vi "DecayAnalysis.vi"() -> ()   [LabVIEW 2015]
uses:
  <vilib>/gmath/SpecialFunctions.llb/Factorial.vi
  <vilib>/Utility/file.llb/Read Delimited Spreadsheet (DBL).vi
  <vilib>/imath/engines/lvmath2/RunTimeEngine/Managers/WorkSpace/UID Generator.vi
  <vilib>/imath/engines/lvmath2/RunTimeEngine/BuiltInFunctions/length/NIMS_length(GM).vi
  <instcachedir>/0/NIMS_length(GM)_47CEC356FCE0482D9BA47DC61C99F2C7.lvgen/NIMS_length(GM)_47CEC356FCE0482D9BA47DC61C99F2C7_000.vi
  <vilib>/imath/engines/lvmath2/RunTimeEngine/RangeToken/NIMS_Range.vi
  <instcachedir>/0/NIMS_Range_D919CC09935940E88F755EC1C6F49AC1.lvgen/NIMS_Range_D919CC09935940E88F755EC1C6F49AC1_001.vi
  <vilib>/imath/engines/lvmath2/RunTimeEngine/RunTimeType/NIMS_RunTimeType_From StrictType (excl LVString).vi
  <instcachedir>/0/NIMS_RunTimeType_From StrictType (excl LVString)_EB1C38A9BC5048DA9ABDA8F781E54D21.lvgen/NIMS_RunTimeType_From StrictType (excl LVString)_EB1C38A9BC5048DA9ABDA8F781E54D21_000.vi
  <vilib>/imathl/engines/lvmath/Functions/Error Handling/Create Error.vi
  <vilib>/imath/engines/lvmath2/RunTimeEngine/LocalVariableDefStatement/MC_LocalVariableDefStatement_Display.vi
  <vilib>/imath/engines/lvmath2/RunTimeEngine/Managers/SymbolTable/Clear UID.vi
  <vilib>/imath/engines/lvmath2/RunTimeEngine/NodeEndStatement/NIMS_NodeEndStatement_Output.vi
  <instcachedir>/0/NIMS_NodeEndStatement_Output_53EC0D466D134D7ABD903AC30B43404B.lvgen/NIMS_NodeEndStatement_Output_53EC0D466D134D7ABD903AC30B43404B_004.vi
  <vilib>/imath/engines/lvmath2/RunTimeEngine/ErrorHandling/NIMS_Finalize Error.vi
  <instcachedir>/0/NIMS_NodeEndStatement_Output_53EC0D466D134D7ABD903AC30B43404B.lvgen/NIMS_NodeEndStatement_Output_53EC0D466D134D7ABD903AC30B43404B_005.vi
  <vilib>/imath/engines/lvmath2/RunTimeEngine/Managers/SymbolTable/NIMS_WorkSpace.lvlib
  <vilib>/Analysis/NI_AALBase.lvlib
  <vilib>/gmath/NI_Gmath.lvlib
panel:
  out "XY Graph 2":cluster{"X Values":dbl[], "y":dbl[]}[](graph)=[{"X Values"=[1.8, 5.4, 9.0, 12.6, 16.2, 19.8, 23.4, 27.0, 30.6, 34.2, 37.8, 41.4, 45.0, 48.6, 52.2, 55.8, 59.4, 63.0, 66.6, 70.2], "y"=[1.0, 0.0, 0.0, 0.0, 0.0, 0.0, 0.0, 0.0, 0.0, 3.0, 11.0, 31.0, 36.0, 61.0, 51.0, 51.0, 35.0, 12.0, 6.0, 3.0]}, {"X Values"=[30.0, 31.0, 32.0, 33.0, 34.0, 35.0, 36.0, 37.0, 38.0, 39.0, 40.0, 41.0, 42.0, 43.0, 44.0, 45.0, 46.0, 47.0, 48.0, 49.0, 50.0, 51.0, 52.0, 53.0, 54.0, 55.0, 56.0, 57.0, 58.0, 59.0, 60.0, 61.0, 62.0, 63.0, 64.0, 65.0, 66.0, 67.0, 68.0, 69.0, 70.0, 71.0, 72.0, 73.0, 74.0, 75.0], "y"=[0.2988606313000329, 0.5013146073419906, 0.8146362369307348, 1.2836692218302488, 1.9632588098580277, 2.916841660360498, 4.213215731631831, 5.921276163374466, 8.102798960407162, 10.80373194720955, 14.044851531372414, 17.81298243003331, 22.054168722898382, 26.670157525365486, 31.519277075431937, 36.422275731610235, 41.17300734877679, 45.55311451354027, 49.349207389668635, 52.370587433934055, 54.46541093129141, 55.53336016523831, 55.53336016523831, 54.485560916837585, 52.467577179176935, 49.605709333040004, 46.062444380680006, 42.02187908412913, 37.67478814439164, 33.20489802556551, 28.777578288823435, 24.53170608227572, 20.57497929481189, 16.982522592543145, 13.798299606441311, 11.03863968515305, 8.697110054969068, 6.749995863558084, 5.161761542720885, 3.8900231916157404, 2.889731513771693, 2.1164230805088455, 1.5285277803674993, 1.0888143093028764, 0.7651127578885076, 0.5304781788026988]}]
  in  "file path (dialog if empty) 2":path=path "C:/Users/jamism2/Desktop/PHYS434jampet/week8/constant.txt"
  out "Results":T1={"Array[0]"=67.95538478705842, "Decay Time  (s)"=137.37711750375104, "Array[2]"=-5.05656305145657, "Array[3]"=0.0, "Array[4]"=0.0, "Array[5]"=0.0, "Array[6]"=0.0, "Array[7]"=0.0, "Array[8]"=0.0}
  in  "file path (dialog if empty)":path=path "C:/Users/jamism2/Desktop/PHYS434jampet/week8/decay.txt"
  out "XY Graph":cluster{"Array":dbl[], "all rows":dbl[]}[](graph)=[{"Array"=[0.0, 1.0, 2.0, 3.0, 4.0, 5.0, 6.0, 7.0, 8.0, 9.0, 10.0, 11.0, 12.0, 13.0, 14.0, 15.0, 16.0, 17.0, 18.0, 19.0, 20.0, 21.0, 22.0, 23.0, 24.0, 25.0, 26.0, 27.0, 28.0, 29.0, 30.0, 31.0, 32.0, 33.0, 34.0, 35.0, 36.0, 37.0, 38.0, 39.0, 40.0, 41.0, 42.0, 43.0, 44.0, 45.0, 46.0, 47.0, 48.0, 49.0, 50.0, 51.0, 52.0, 53.0, 54.0, 55.0, 56.0, 57.0, 58.0, 59.0, 60.0, 61.0, 62.0, 63.0, 64.0, 65.0, 66.0, 67.0, 68.0, 69.0, 70.0, 71.0, 72.0, 73.0, 74.0, 75.0, 76.0, 77.0, 78.0, 79.0, 80.0, 81.0, 82.0, 83.0, 84.0, 85.0, 86.0, 87.0, 88.0, 89.0, 90.0, 91.0, 92.0, 93.0, 94.0, 95.0, 96.0, 97.0, 98.0, 99.0, 100.0, 101.0, 102.0, 103.0, 104.0, 105.0, 106.0, 107.0, 108.0, 109.0, 110.0, 111.0, 112.0, 113.0, 114.0, 115.0, 116.0, 117.0, 118.0, 119.0, 120.0, 121.0, 122.0, 123.0, 124.0, 125.0, 126.0, 127.0, 128.0, 129.0, 130.0, 131.0, 132.0, 133.0, 134.0, 135.0, 136.0, 137.0, 138.0, 139.0, 140.0, 141.0, 142.0, 143.0, 144.0, 145.0, 146.0, 147.0, 148.0, 149.0, 150.0, 151.0, 152.0, 153.0, 154.0, 155.0, 156.0, 157.0, 158.0, 159.0, 160.0, 161.0, 162.0, 163.0, 164.0, 165.0, 166.0, 167.0, 168.0, 169.0, 170.0, 171.0, 172.0, 173.0, 174.0, 175.0, 176.0, 177.0, 178.0, 179.0, 180.0, 181.0, 182.0, 183.0, 184.0, 185.0, 186.0, 187.0, 188.0, 189.0, 190.0, 191.0, 192.0, 193.0, 194.0, 195.0, 196.0, 197.0, 198.0, 199.0, 200.0, 201.0, 202.0, 203.0, 204.0, 205.0, 206.0, 207.0, 208.0, 209.0, 210.0, 211.0, 212.0, 213.0, 214.0, 215.0, 216.0, 217.0, 218.0, 219.0, 220.0, 221.0, 222.0, 223.0, 224.0, 225.0, 226.0, 227.0, 228.0, 229.0, 230.0, 231.0, 232.0, 233.0, 234.0, 235.0, 236.0, 237.0, 238.0, 239.0, 240.0, 241.0, 242.0, 243.0, 244.0, 245.0, 246.0, 247.0, 248.0, 249.0, 250.0, 251.0, 252.0, 253.0, 254.0, 255.0, 256.0, 257.0, 258.0, 259.0, 260.0, 261.0, 262.0, 263.0, 264.0, 265.0, 266.0, 267.0, 268.0, 269.0, 270.0, 271.0, 272.0, 273.0, 274.0, 275.0, 276.0, 277.0, 278.0, 279.0, 280.0, 281.0, 282.0, 283.0, 284.0, 285.0, 286.0, 287.0, 288.0, 289.0, 290.0, 291.0, 292.0, 293.0, 294.0, 295.0, 296.0, 297.0, 298.0, 299.0, 300.0, 301.0], "all rows"=[0.0, 47.0, 44.0, 50.0, 68.0, 51.0, 62.0, 72.0, 48.0, 45.0, 45.0, 74.0, 55.0, 72.0, 61.0, 65.0, 59.0, 55.0, 73.0, 56.0, 57.0, 63.0, 54.0, 59.0, 53.0, 55.0, 54.0, 50.0, 53.0, 50.0, 43.0, 50.0, 47.0, 45.0, 43.0, 52.0, 68.0, 50.0, 40.0, 55.0, 62.0, 42.0, 53.0, 55.0, 60.0, 50.0, 51.0, 42.0, 48.0, 35.0, 51.0, 33.0, 35.0, 43.0, 43.0, 54.0, 44.0, 35.0, 31.0, 42.0, 39.0, 46.0, 39.0, 42.0, 41.0, 52.0, 34.0, 42.0, 45.0, 40.0, 50.0, 38.0, 42.0, 30.0, 48.0, 34.0, 27.0, 36.0, 39.0, 32.0, 33.0, 36.0, 26.0, 31.0, 35.0, 25.0, 23.0, 25.0, 38.0, 26.0, 32.0, 34.0, 31.0, 25.0, 36.0, 27.0, 28.0, 26.0, 28.0, 34.0, 30.0, 28.0, 23.0, 30.0, 19.0, 29.0, 17.0, 16.0, 19.0, 24.0, 22.0, 19.0, 27.0, 18.0, 20.0, 23.0, 28.0, 29.0, 28.0, 29.0, 31.0, 21.0, 25.0, 28.0, 26.0, 19.0, 22.0, 27.0, 21.0, 14.0, 9.0, 20.0, 21.0, 15.0, 15.0, 18.0, 15.0, 18.0, 14.0, 14.0, 13.0, 13.0, 12.0, 26.0, 21.0, 26.0, 21.0, 12.0, 7.0, 20.0, 11.0, 18.0, 12.0, 12.0, 16.0, 12.0, 19.0, 13.0, 9.0, 15.0, 14.0, 10.0, 14.0, 13.0, 13.0, 16.0, 12.0, 22.0, 16.0, 17.0, 18.0, 11.0, 16.0, 5.0, 7.0, 9.0, 15.0, 9.0, 13.0, 14.0, 8.0, 10.0, 12.0, 10.0, 17.0, 14.0, 13.0, 12.0, 10.0, 11.0, 9.0, 9.0, 8.0, 19.0, 7.0, 19.0, 10.0, 8.0, 8.0, 15.0, 11.0, 15.0, 14.0, 9.0, 11.0, 10.0, 8.0, 8.0, 7.0, 9.0, 4.0, 12.0, 8.0, 4.0, 6.0, 10.0, 7.0, 18.0, 4.0, 6.0, 9.0, 5.0, 16.0, 4.0, 8.0, 7.0, 6.0, 9.0, 3.0, 8.0, 4.0, 7.0, 4.0, 4.0, 13.0, 7.0, 10.0, 7.0, 10.0, 8.0, 5.0, 3.0, 6.0, 11.0, 4.0, 5.0, 5.0, 6.0, 11.0, 2.0, 5.0, 6.0, 4.0, 12.0, 7.0, 7.0, 6.0, 13.0, 5.0, 4.0, 2.0, 7.0, 3.0, 7.0, 5.0, 6.0, 9.0, 2.0, 5.0, 0.0, 6.0, 7.0, 6.0, 9.0, 7.0, 4.0, 4.0, 5.0, 2.0, 6.0, 3.0, 6.0, 7.0, 6.0, 6.0, 7.0, 4.0, 7.0, 5.0, 8.0, 5.0, 7.0, 7.0, 10.0, 2.0, 3.0, 8.0, 5.0, 2.0, 11.0, 3.0]}, {"Array"=[0.0, 1.0, 2.0, 3.0, 4.0, 5.0, 6.0, 7.0, 8.0, 9.0, 10.0, 11.0, 12.0, 13.0, 14.0, 15.0, 16.0, 17.0, 18.0, 19.0, 20.0, 21.0, 22.0, 23.0, 24.0, 25.0, 26.0, 27.0, 28.0, 29.0, 30.0, 31.0, 32.0, 33.0, 34.0, 35.0, 36.0, 37.0, 38.0, 39.0, 40.0, 41.0, 42.0, 43.0, 44.0, 45.0, 46.0, 47.0, 48.0, 49.0, 50.0, 51.0, 52.0, 53.0, 54.0, 55.0, 56.0, 57.0, 58.0, 59.0, 60.0, 61.0, 62.0, 63.0, 64.0, 65.0, 66.0, 67.0, 68.0, 69.0, 70.0, 71.0, 72.0, 73.0, 74.0, 75.0, 76.0, 77.0, 78.0, 79.0, 80.0, 81.0, 82.0, 83.0, 84.0, 85.0, 86.0, 87.0, 88.0, 89.0, 90.0, 91.0, 92.0, 93.0, 94.0, 95.0, 96.0, 97.0, 98.0, 99.0, 100.0, 101.0, 102.0, 103.0, 104.0, 105.0, 106.0, 107.0, 108.0, 109.0, 110.0, 111.0, 112.0, 113.0, 114.0, 115.0, 116.0, 117.0, 118.0, 119.0, 120.0, 121.0, 122.0, 123.0, 124.0, 125.0, 126.0, 127.0, 128.0, 129.0, 130.0, 131.0, 132.0, 133.0, 134.0, 135.0, 136.0, 137.0, 138.0, 139.0, 140.0, 141.0, 142.0, 143.0, 144.0, 145.0, 146.0, 147.0, 148.0, 149.0, 150.0, 151.0, 152.0, 153.0, 154.0, 155.0, 156.0, 157.0, 158.0, 159.0, 160.0, 161.0, 162.0, 163.0, 164.0, 165.0, 166.0, 167.0, 168.0, 169.0, 170.0, 171.0, 172.0, 173.0, 174.0, 175.0, 176.0, 177.0, 178.0, 179.0, 180.0, 181.0, 182.0, 183.0, 184.0, 185.0, 186.0, 187.0, 188.0, 189.0, 190.0, 191.0, 192.0, 193.0, 194.0, 195.0, 196.0, 197.0, 198.0, 199.0, 200.0, 201.0, 202.0, 203.0, 204.0, 205.0, 206.0, 207.0, 208.0, 209.0, 210.0, 211.0, 212.0, 213.0, 214.0, 215.0, 216.0, 217.0, 218.0, 219.0, 220.0, 221.0, 222.0, 223.0, 224.0, 225.0, 226.0, 227.0, 228.0, 229.0, 230.0, 231.0, 232.0, 233.0, 234.0, 235.0, 236.0, 237.0, 238.0, 239.0, 240.0, 241.0, 242.0, 243.0, 244.0, 245.0, 246.0, 247.0, 248.0, 249.0, 250.0, 251.0, 252.0, 253.0, 254.0, 255.0, 256.0, 257.0, 258.0, 259.0, 260.0, 261.0, 262.0, 263.0, 264.0, 265.0, 266.0, 267.0, 268.0, 269.0, 270.0, 271.0, 272.0, 273.0, 274.0, 275.0, 276.0, 277.0, 278.0, 279.0, 280.0, 281.0, 282.0, 283.0, 284.0, 285.0, 286.0, 287.0, 288.0, 289.0, 290.0, 291.0, 292.0, 293.0, 294.0, 295.0, 296.0, 297.0, 298.0, 299.0, 300.0, 301.0], "all rows"=[62.89882173560185, 62.40595470267312, 61.91666233734299, 61.43091871325081, 60.94869809207474, 60.46997492216793, 59.99472383720457, 59.52291965483585, 59.05453737535557, 58.58955218037546, 58.127939431510164, 57.669674669071675, 57.21473361077329, 56.763092150442944, 56.31472635674591, 55.8696124719167, 55.427726910500255, 54.989046258102164, 54.553547270148, 54.121206870651676, 53.692002150992685, 53.265910368702244, 52.84290894625819, 52.42297546988873, 52.00608768838473, 51.59222351192068, 51.18136101088424, 50.77347841471423, 50.36855411074709, 49.966566643071616, 49.567494711392115, 49.17131716989979, 48.77801302615216, 48.38756143996086, 47.999941722287296, 47.61513333414638, 47.233115885518245, 46.85386913426785, 46.47737298507236, 46.103607488356346, 45.73255283923475, 45.36418937646343, 44.99849758139739, 44.63545807695652, 44.27505162659887, 43.91725913330131, 43.562061638547696, 43.209440321324266, 42.859376497122355, 42.51185161694836, 42.16684726634089, 41.824345164395005, 41.4843271627936, 41.14677524484569, 40.811671524531874, 40.47899824555646, 40.148737780406734, 39.820872629418815, 39.49538541985047, 39.172258904960536, 38.851475963095076, 38.53301959678013, 38.21687293182107, 37.903019216408495, 37.59144182023058, 37.282124233591865, 36.975050066538465, 36.67020304798963, 36.36756702487551, 36.06712596128133, 35.76886393759764, 35.47276514967678, 35.17881390799547, 34.886994636823445, 34.59729187339815, 34.30969026710541, 34.02417457866603, 33.7407296793283, 33.45934055006637, 33.17999228078446, 32.902670069526735, 32.62735922169306, 32.35404514926033, 32.08271337000952, 31.813349506758264, 31.54593928659908, 31.280468540143097, 31.0169232007692, 30.75528930387872, 30.495552986155495, 30.237700484831237, 29.981718136956317, 29.7275923786758, 29.475309744510717, 29.224856866644565, 28.976220474214983, 28.72938739261057, 28.48434454277278, 28.24107894050291, 27.9995776957741, 27.759828012048303, 27.521817185598266, 27.285532604834344, 27.050961749636294, 26.818092190689818, 26.586911588828013, 26.357407694377507, 26.129568346509412, 25.903381472594923, 25.678835087565652, 25.45591729327854, 25.23461627788543, 25.014920315207164, 24.796817764112262, 24.580297067900077, 24.365346753688442, 24.151955431805735, 23.940111795187388, 23.729804618776754, 23.521022758930304, 23.313755152827163, 23.10799081788292, 22.90371885116769, 22.70092842882839, 22.499608805515216, 22.29974931381227, 22.101339363672317, 21.90436844185566, 21.708826111373057, 21.514702010932695, 21.32198585439117, 21.130667430208447, 20.940736600906796, 20.752183302533602, 20.564997544128133, 20.379169407192112, 20.194689045164196, 20.011546682898196, 19.829732616145147, 19.6492372110391, 19.470050903586607, 19.292164199160023, 19.115567671994338, 18.94025196468778, 18.76620778770596, 18.593425918889658, 18.42189720296615, 18.25161255106413, 18.082562940232055, 17.914739412960095, 17.748133076705464, 17.58273510342125, 17.41853672908862, 17.255529253252448, 17.093704038560286, 16.93305251030473, 16.773566155969014, 16.615236524775998, 16.458055227240354, 16.30201393472405, 16.14710437899502, 15.993318351789057, 15.840647704374891, 15.689084347122378, 15.538620249073883, 15.38924743751872, 15.240957997570714, 15.093744071748787, 14.947597859560638, 14.802511617089394, 14.65847765658329, 14.515488346048311, 14.373536108843794, 14.23261342328096, 14.092712822224353, 13.953826892696188, 13.815948275483546, 13.679069664748429, 13.543183807640652, 13.408283503913516, 13.2743616055423, 13.14141101634549, 13.009424691608803, 12.87839563771185, 12.748316911757627, 12.619181621204572, 12.490982923501381, 12.36371402572442, 12.23736818421781, 12.11193870423606, 11.987418939589372, 11.863802292291432, 11.741082212209847, 11.619252196719014, 11.49830579035563, 11.378236584476564, 11.259038216919343, 11.140704371664974, 11.023228778503338, 10.906605212700896, 10.790827494670879, 10.675889489645854, 10.561785107352637, 10.448508301689603, 10.336053070406319, 10.22441345478548, 10.113583539327191, 10.003557451435515, 9.894329361107303, 9.785893480623255, 9.678244064241273, 9.571375407891995, 9.46528184887655, 9.359957765566506, 9.255397577105995, 9.151595743116005, 9.048546763400786, 8.946245177656454, 8.844685565181603, 8.743862544590133, 8.643770773526057, 8.544404948380471, 8.445759804010468, 8.347830113460219, 8.25061068768396, 8.154096375271056, 8.058282062173042, 7.963162671432644, 7.86873316291475, 7.774988533039367, 7.681923814516474, 7.589534076082836, 7.497814422240688, 7.406759992998361, 7.3163659636127365, 7.226627544333618, 7.137539980149916, 7.049098550537711, 6.9612985692101015, 6.874135383868917, 6.7876043759581774, 6.70170096041939, 6.616420585448581, 6.531758732255121, 6.447710914822276, 6.364272679669516, 6.281439605616515, 6.199207303548913, 6.1175714161857195, 6.036527617848459, 5.956071614231935, 5.876199142176717, 5.796905969443221, 5.71818789448747, 5.640040746238449, 5.562460383877114, 5.485442696616951, 5.408983603486189, 5.333079053111526, 5.257725023503485, 5.18291752184328, 5.108652584271259, 5.034926275676859, 4.961734689490105, 4.889073947474597, 4.816940199522031, 4.745329623448174, 4.6742384247903415, 4.603662836606348, 4.53359911927489, 4.46404356029741, 4.394992474101362, 4.326442201844938, 4.258389111223191, 4.190829596275566, 4.123760077194826, 4.057177000137375, 3.9910768370349468, 3.9254560854076592, 3.8603112681784255, 3.7956389334887097, 3.731435654515642, 3.667698029290409, 3.6044226805180175, 3.54160625539832, 3.479245425448382, 3.4173368863260896, 3.3558773576550793, 3.294863582850902, 3.2342923289484906, 3.174160386430823, 3.114464569058881, 3.0552017137027976, 2.996368680174288, 2.9379623510602153, 2.8799796315574318, 2.8224174493087864, 2.765272754240339, 2.7085425183997263, 2.6522237357957286, 2.596313422238988, 2.540808615183895]}]
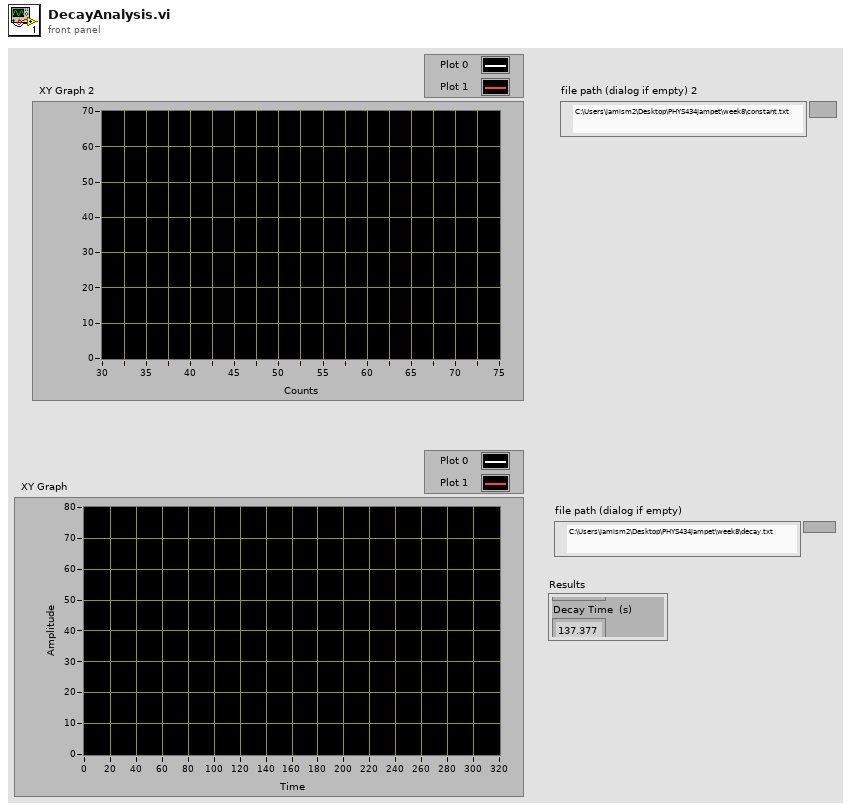
[diagram p1: front panel]
types:
  T1 = cluster{"Array[0]":dbl, "Decay Time  (s)":dbl, "Array[2]":dbl, "Array[3]":dbl, "Array[4]":dbl, "Array[5]":dbl, "Array[6]":dbl, "Array[7]":dbl, "Array[8]":dbl}
  T2 = cluster{"X Values":dbl[], "Histogram: h(x)":i32[]}
  T3 = cluster{"Array[0]":dbl, "Array[1]":dbl, "Array[2]":dbl, "Array[3]":dbl, "Array[4]":dbl, "Array[5]":dbl, "Array[6]":dbl, "Array[7]":dbl, "Array[8]":dbl}
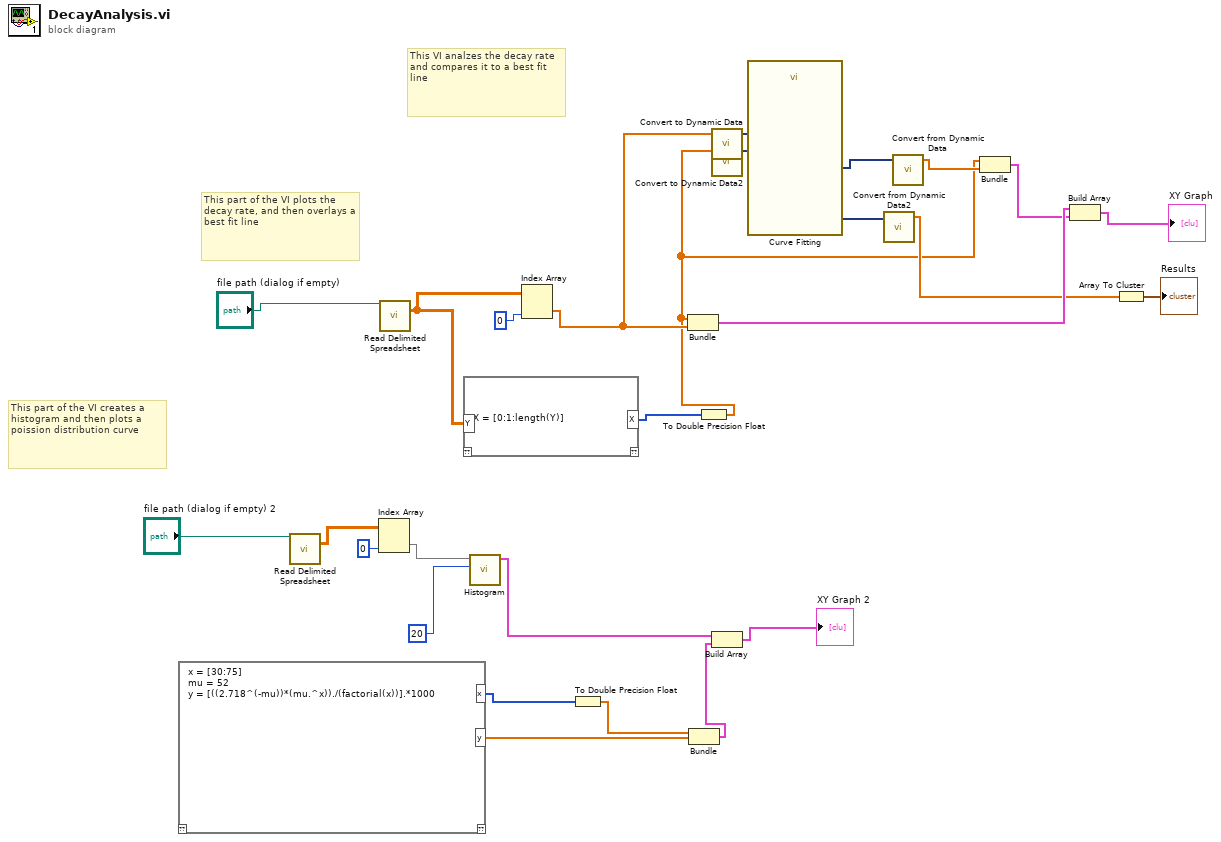
[diagram p0: block diagram]
diagram:
  # "This part of the VI plots the decay rate, and then overlays a best fit line"
  # "This part of the VI creates a histogram and then plots a poission distribution curve"
  # "This VI analzes the decay rate and compares it to a best fit line"
  n1 = mathscript code="x = [30:75]\nmu = 52\ny = [((2.718^(-mu))*(mu.^x))./(factorial(x))].*1000"() -> ("y"=w4:dbl[], "x"=w6:i32[])  [unwired: 1 in, 1 out]
  n2 = call-poly <vilib>:"Read Delimited Spreadsheet.vi"("file path (dialog if empty)"="file path (dialog if empty) 2") -> ("all rows"=w10:dbl[][])  [unwired: 9 in, 5 out]
  n3 = Index Array(array=w10, index (col)=0 ("disabled index (col)")) -> (element=w8:dbl[])  [unwired: 1 in]
  n4 = call-poly <vilib>:"Read Delimited Spreadsheet.vi"("file path (dialog if empty)"="file path (dialog if empty)") -> ("all rows"=w25:dbl[][])  [unwired: 9 in, 5 out]
  n5 = mathscript code="X = [0:1:length(Y)]"("Y"=w25) -> ("X"=w24:i32[])  [unwired: 1 in, 1 out]
  n6 = call <vilib>:"Histogram.vi"("intervals"=20, "X"=w8) -> ("Histogram Graph"=w2:T2)  [unwired: 6 in, 3 out]
  n7 = Index Array(array=w25, index (col)=0 ("disabled index (col)")) -> (element=w23:dbl[])  [unwired: 1 in]
  n8 = To Double Precision Float(number=w6) -> (double precision float=w5:dbl[])
  n9 = Bundle(w5, "y"=w4) -> (w3:cluster{dbl[], "y":dbl[]})  [unwired: 1 in]
  n10 = To Double Precision Float(number=w24) -> (double precision float=w7:dbl[])
  n11 = Bundle(w7, "all rows"=w23) -> (w19:cluster{dbl[], "all rows":dbl[]})  [unwired: 1 in]
  n12 = call "Convert to Dynamic Data"("Array"=w23) -> ("Dynamic Data Type"=w22:dynamicdata)  [unwired: 3 in]
  n13 = call "Convert to Dynamic Data2"("Array"=w7) -> ("Dynamic Data Type"=w21:dynamicdata)  [unwired: 3 in]
  n14 = Build Array(w2, w3) -> (→"XY Graph 2":cluster{"X Values":dbl[], "y":dbl[]}[])
  n15 = call "Curve Fitting"("Locations"=w21, "Signals"=w22) -> ("best fit"=w20:dynamicdata, "non-linear coefficients"=w15:dynamicdata)  [unwired: 5 in, 3 out]
  n16 = call "Convert from Dynamic Data2"("Dynamic Data Type"=w15) -> ("Array"=w14:dbl[])  [unwired: 3 in]
  n17 = call "Convert from Dynamic Data"("Dynamic Data Type"=w20) -> ("Array"=w16:dbl[])  [unwired: 3 in]
  n18 = Bundle(w7, "Array"=w16) -> (w18:cluster{dbl[], "Array":dbl[]})  [unwired: 1 in]
  n19 = Build Array(w19, w18) -> (→"XY Graph":cluster{dbl[], "Array":dbl[]}[])
  n20 = Array To Cluster(array=w14) -> (cluster=→"Results":T3)
